vi "Slide Servo home.vi"(8 "error in":errorcluster, 10 "NewVal":bool) -> (0 "error out":errorcluster)   [LabVIEW 2015]
uses:
  Galobal variable_TI.vi
  Project Setup/Globle Variable/GR_Servo.vi
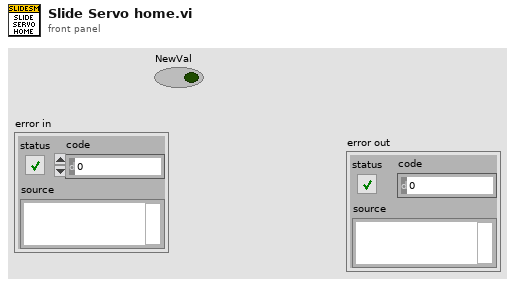
[diagram p1: front panel]
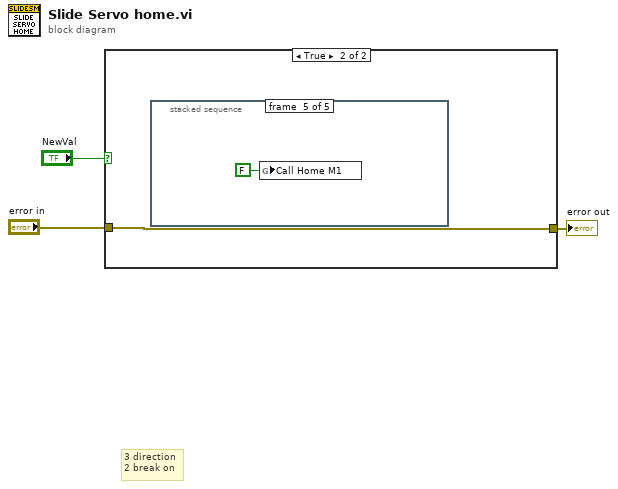
[diagram p0: block diagram]
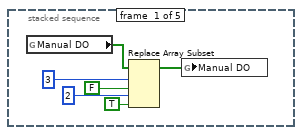
[diagram p3: hidden frame]
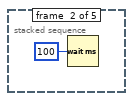
[diagram p4: hidden frame]
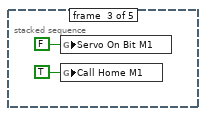
[diagram p5: hidden frame]
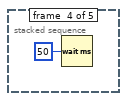
[diagram p6: hidden frame]
diagram:
  # "3 direction\n2 break on"
  n1 = case shown="True" "NewVal" {
    tunnel: "error in" -> [w4 w5]
    tunnel: [w4 w5] -> w1
    frame False {
    }
    frame True {
      n2 = stacked-sequence {
        frame #0 {
          n3 = global read "Galobal variable_TI.vi" "Manual DO"() -> (w7:bool[])
          n4 = Replace Array Subset(array=w7, new element #1=FALSE ("new element/subarray"), index #1=3 ("index"), new element #2=TRUE ("new element/subarray"), index #2=2 ("index")) -> (w11:bool[])
          n5 = global write "Galobal variable_TI.vi" "Manual DO"(w11) -> ()
        }
        frame #1 {
          n6 = Wait (ms)(milliseconds to wait=u32 100) -> ()  [unwired: 1 out]
        }
        frame #2 {
          n7 = global write "GR_Servo.vi" "Servo On Bit M1"(FALSE ("Servo On Bit")) -> ()
          n8 = global write "Galobal variable_TI.vi" "Call Home M1"(TRUE ("Call Home M1")) -> ()
        }
        frame #3 {
          n9 = Wait (ms)(milliseconds to wait=u32 50) -> ()  [unwired: 1 out]
        }
        frame #4 {
          n10 = global write "Galobal variable_TI.vi" "Call Home M1"(FALSE ("Call Home M1")) -> ()
        }
      }
    }
  }
  "error out" <- w1
